vi "read_NP_Dop.vi"() -> (0 "P_Dop Active":bool, 1 "P_Dop Bubbler":bool, 2 "P_Dop Run":bool, 3 "P_Dop H2 Dilute":bool, 4 "P_Dop Gas Source":bool, 5 "P_Dop Remote":bool, 6 "N/P_Dop Flow 1":dbl, 7 "N/P Dopant DA Switch":bool, 8 "N/P_Dop Flow 2 or 4":dbl, 10 "N/P_Dop Flow 3":dbl, 14 "N_Dop Active":bool, 15 "N_Dop Bubbler":bool, 16 "N_Dop Run":bool, 17 "N_Dop H2 Dilute":bool, 18 "N_Dop Gas Source":bool, 19 "N_Dop Remote":bool)   [LabVIEW 2011]
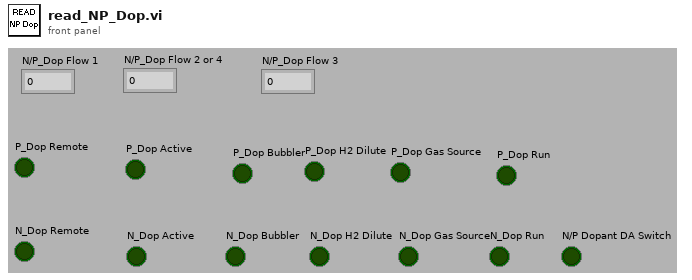
[diagram p1: front panel]
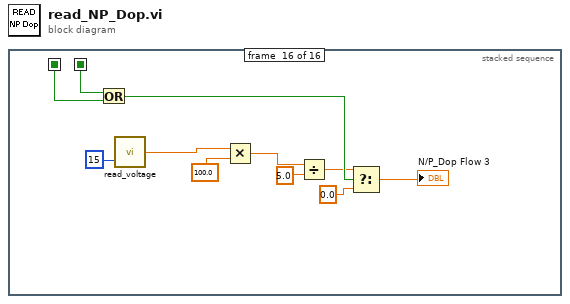
[diagram p0: block diagram]
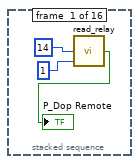
[diagram p2: hidden frame]
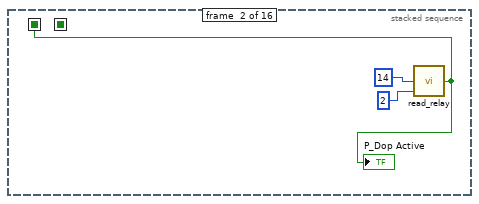
[diagram p3: hidden frame]
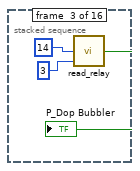
[diagram p4: hidden frame]
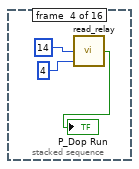
[diagram p5: hidden frame]
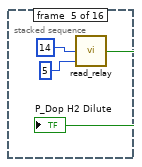
[diagram p6: hidden frame]
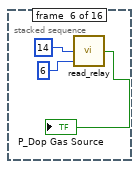
[diagram p7: hidden frame]
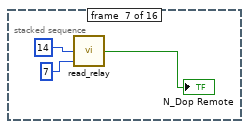
[diagram p8: hidden frame]
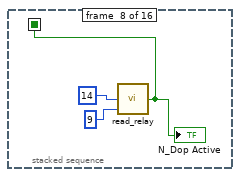
[diagram p9: hidden frame]
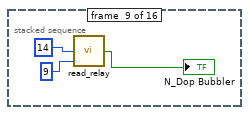
[diagram p10: hidden frame]
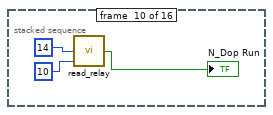
[diagram p11: hidden frame]
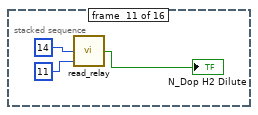
[diagram p12: hidden frame]
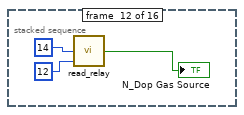
[diagram p13: hidden frame]
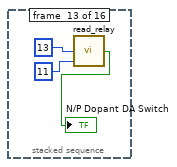
[diagram p14: hidden frame]
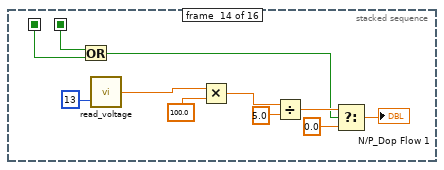
[diagram p15: hidden frame]
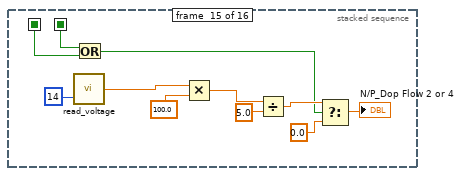
[diagram p16: hidden frame]
diagram:
  n1 = stacked-sequence {
    seq-local: [_ w4 _ _ _ _ _ _ _ _ _ _ _ _ _ _] -> [_ _ _ _ _ _ _ _ _ _ _ _ _ w44 w52 w66]
    seq-local: [_ _ _ _ _ _ _ w22 _ _ _ _ _ _ _ _] -> [_ _ _ _ _ _ _ _ _ _ _ _ _ w45 w53 w67]
    frame #0 {
      n2 = call "read_relay.vi"("Relay"=1, "Slot"=14) -> ("Relay Status"=→"P_Dop Remote":bool)  [unwired: 1 out]
    }
    frame #1 {
      n3 = call "read_relay.vi"("Relay"=2, "Slot"=14) -> ("Relay Status"=w4:bool)  [unwired: 1 out]
      "P_Dop Active" <- w4
    }
    frame #2 {
      n4 = call "read_relay.vi"("Relay"=3, "Slot"=14) -> ("Relay Status"=→"P_Dop Bubbler":bool)  [unwired: 1 out]
    }
    frame #3 {
      n5 = call "read_relay.vi"("Relay"=4, "Slot"=14) -> ("Relay Status"=→"P_Dop Run":bool)  [unwired: 1 out]
    }
    frame #4 {
      n6 = call "read_relay.vi"("Relay"=5, "Slot"=14) -> ("Relay Status"=→"P_Dop H2 Dilute":bool)  [unwired: 1 out]
    }
    frame #5 {
      n7 = call "read_relay.vi"("Relay"=6, "Slot"=14) -> ("Relay Status"=→"P_Dop Gas Source":bool)  [unwired: 1 out]
    }
    frame #6 {
      n8 = call "read_relay.vi"("Relay"=7, "Slot"=14) -> ("Relay Status"=→"N_Dop Remote":bool)  [unwired: 1 out]
    }
    frame #7 {
      n9 = call "read_relay.vi"("Relay"=9, "Slot"=14) -> ("Relay Status"=w22:bool)  [unwired: 1 out]
      "N_Dop Active" <- w22
    }
    frame #8 {
      n10 = call "read_relay.vi"("Relay"=9, "Slot"=14) -> ("Relay Status"=→"N_Dop Bubbler":bool)  [unwired: 1 out]
    }
    frame #9 {
      n11 = call "read_relay.vi"("Relay"=10, "Slot"=14) -> ("Relay Status"=→"N_Dop Run":bool)  [unwired: 1 out]
    }
    frame #10 {
      n12 = call "read_relay.vi"("Relay"=11, "Slot"=14) -> ("Relay Status"=→"N_Dop H2 Dilute":bool)  [unwired: 1 out]
    }
    frame #11 {
      n13 = call "read_relay.vi"("Relay"=12, "Slot"=14) -> ("Relay Status"=→"N_Dop Gas Source":bool)  [unwired: 1 out]
    }
    frame #12 {
      n14 = call "read_relay.vi"("Relay"=11, "Slot"=13) -> ("Relay Status"=→"N/P Dopant DA Switch":bool)  [unwired: 1 out]
    }
    frame #13 {
      n15 = Or(x=w45, y=w44) -> (x .or. y?=w41:bool)
      n16 = call "read_voltage.vi"("Channel"=13) -> ("Voltage"=w46:dbl)  [unwired: 1 in]
      n17 = Multiply(x=w46, y=100.0) -> (x*y=w48:dbl)
      n18 = Divide(x=w48, y=5.0) -> (x/y=w43:dbl)
      n19 = Select(t=w43, s=w41, f=0.0) -> (s? t:f=→"N/P_Dop Flow 1":dbl)
    }
    frame #14 {
      n20 = call "read_voltage.vi"("Channel"=14) -> ("Voltage"=w61:dbl)  [unwired: 1 in]
      n21 = Or(x=w53, y=w52) -> (x .or. y?=w51:bool)
      n22 = Multiply(x=w61, y=100.0) -> (x*y=w59:dbl)
      n23 = Divide(x=w59, y=5.0) -> (x/y=w56:dbl)
      n24 = Select(t=w56, s=w51, f=0.0) -> (s? t:f=→"N/P_Dop Flow 2 or 4":dbl)
    }
    frame #15 {
      n25 = Or(x=w67, y=w66) -> (x .or. y?=w65:bool)
      n26 = call "read_voltage.vi"("Channel"=15) -> ("Voltage"=w68:dbl)  [unwired: 1 in]
      n27 = Multiply(x=w68, y=100.0) -> (x*y=w70:dbl)
      n28 = Divide(x=w70, y=5.0) -> (x/y=w64:dbl)
      n29 = Select(t=w64, s=w65, f=0.0) -> (s? t:f=→"N/P_Dop Flow 3":dbl)
    }
  }
